vi "Jarvis main.vi"() -> ()   [LabVIEW 2017]
uses:
  SSL Referee Game Status.ctl
  Filters/Estimadores.ctl
  Control/SSL Data Control.ctl
  Control/SSL UDP Address.ctl
  Control/File Player.ctl
  Intel/Command Enum.ctl
  DrawTargets.ctl
  Util/Events/Events.ctl
  passTestStates.ctl
  SSL/SSL Field State.ctl
  SSL Detection Frame.ctl
  SSL Detection Robot.ctl
  <vilib>/Analysis/Matrix/Datatypes/RealMatrix.ctl
  SSL Detection Ball.ctl
  <extravilib>/ChannelInstances/Lossy Stream-a[.](u8)/Read With Abort.vi
  <extravilib>/ChannelInstances/Lossy Stream-t'SSL Referee Game Status.ctl'/Write With Abort.vi
  <extravilib>/ChannelInstances/Lossy Stream-c(a[.](c(c(dbl,dbl,dbl,dbl,dbl),c(dbl,dbl,dbl,dbl,dbl),c(dbl,dbl,dbl,dbl,dbl,u32),u32,u32)),t'Events.ctl')/Write With Abort.vi
  <extravilib>/ChannelInstances/Lossy Stream-c(t'AI Ball.ctl',a[.](c(c(dbl,dbl,dbl,dbl,dbl),c(dbl,dbl,dbl,dbl,dbl),c(dbl,dbl,dbl,dbl,dbl,u32),u32,u32)))/Write With Abort.vi
  <extravilib>/ChannelInstances/Lossy Stream-t'AI Input.ctl'/Read With Abort.vi
  <extravilib>/ChannelInstances/Lossy Stream-t'SSL Field State.ctl'/Write With Abort.vi
  <extravilib>/ChannelInstances/Lossy Stream-c(t'AI Ball.ctl',a[.](c(c(dbl,dbl,dbl,dbl,dbl),c(dbl,dbl,dbl,dbl,dbl),c(dbl,dbl,dbl,dbl,dbl,u32),u32,u32)))/Read With Abort.vi
  <extravilib>/ChannelInstances/Lossy Stream-c(a[.](c(c(dbl,dbl,dbl,dbl,dbl),c(dbl,dbl,dbl,dbl,dbl),c(dbl,dbl,dbl,dbl,dbl,u32),u32,u32)),t'Events.ctl')/Read With Abort.vi
  <extravilib>/ChannelInstances/Lossy Stream-a[.](i32)/Write With Abort.vi
  <extravilib>/ChannelInstances/Lossy Stream-t'SSL Referee Game Status.ctl'/Read With Abort.vi
  <extravilib>/ChannelInstances/Lossy Stream-t'SSL Field State.ctl'/Read With Abort.vi
  <extravilib>/ChannelInstances/Lossy Stream-t'AI Input.ctl'/Write With Abort.vi
  <extravilib>/ChannelInstances/Lossy Stream-a[.](u8)/EndpointRead.vi
  <extravilib>/ChannelInstances/Lossy Stream-t'SSL Referee Game Status.ctl'/Endpoint.vi
  <extravilib>/ChannelInstances/Lossy Stream-c(a[.](c(c(dbl,dbl,dbl,dbl,dbl),c(dbl,dbl,dbl,dbl,dbl),c(dbl,dbl,dbl,dbl,dbl,u32),u32,u32)),t'Events.ctl')/Endpoint.vi
  <extravilib>/ChannelInstances/Lossy Stream-c(t'AI Ball.ctl',a[.](c(c(dbl,dbl,dbl,dbl,dbl),c(dbl,dbl,dbl,dbl,dbl),c(dbl,dbl,dbl,dbl,dbl,u32),u32,u32)))/Endpoint.vi
  <extravilib>/ChannelInstances/Lossy Stream-t'AI Input.ctl'/EndpointRead.vi
  <extravilib>/ChannelInstances/Lossy Stream-t'SSL Field State.ctl'/Endpoint.vi
  <extravilib>/ChannelInstances/Lossy Stream-c(t'AI Ball.ctl',a[.](c(c(dbl,dbl,dbl,dbl,dbl),c(dbl,dbl,dbl,dbl,dbl),c(dbl,dbl,dbl,dbl,dbl,u32),u32,u32)))/EndpointRead.vi
  <extravilib>/ChannelInstances/Lossy Stream-c(a[.](c(c(dbl,dbl,dbl,dbl,dbl),c(dbl,dbl,dbl,dbl,dbl),c(dbl,dbl,dbl,dbl,dbl,u32),u32,u32)),t'Events.ctl')/EndpointRead.vi
  <extravilib>/ChannelInstances/Lossy Stream-a[.](i32)/Endpoint.vi
  <extravilib>/ChannelInstances/Lossy Stream-t'SSL Referee Game Status.ctl'/EndpointRead.vi
  <extravilib>/ChannelInstances/Lossy Stream-t'SSL Field State.ctl'/EndpointRead.vi
  <extravilib>/ChannelInstances/Lossy Stream-t'AI Input.ctl'/Endpoint.vi
  <extravilib>/ChannelInstances/Lossy Stream-t'AI Input.ctl'/Instantiate.vi
  <extravilib>/ChannelInstances/Lossy Stream-t'SSL Field State.ctl'/Instantiate.vi
  <extravilib>/ChannelInstances/Lossy Stream-t'AI Input.ctl'/)Channel.vi
  <resource>/ChannelSupport/_ChannelSupport/WaitIfNeeded.vi
  <extravilib>/ChannelInstances/Lossy Stream-c(t'AI Ball.ctl',a[.](c(c(dbl,dbl,dbl,dbl,dbl),c(dbl,dbl,dbl,dbl,dbl),c(dbl,dbl,dbl,dbl,dbl,u32),u32,u32)))/Instantiate.vi
  <extravilib>/ChannelInstances/Lossy Stream-c(a[.](c(c(dbl,dbl,dbl,dbl,dbl),c(dbl,dbl,dbl,dbl,dbl),c(dbl,dbl,dbl,dbl,dbl,u32),u32,u32)),t'Events.ctl')/Instantiate.vi
  <extravilib>/ChannelInstances/Lossy Stream-a[.](u8)/Instantiate.vi
  <extravilib>/ChannelInstances/Lossy Stream-a[.](u8)/)Channel.vi
  <extravilib>/ChannelInstances/Lossy Stream-c(t'AI Ball.ctl',a[.](c(c(dbl,dbl,dbl,dbl,dbl),c(dbl,dbl,dbl,dbl,dbl),c(dbl,dbl,dbl,dbl,dbl,u32),u32,u32)))/)Channel.vi
  <extravilib>/ChannelInstances/Lossy Stream-c(a[.](c(c(dbl,dbl,dbl,dbl,dbl),c(dbl,dbl,dbl,dbl,dbl),c(dbl,dbl,dbl,dbl,dbl,u32),u32,u32)),t'Events.ctl')/)Channel.vi
  <extravilib>/ChannelInstances/Lossy Stream-a[.](i32)/Instantiate.vi
  <extravilib>/ChannelInstances/Lossy Stream-t'SSL Referee Game Status.ctl'/Instantiate.vi
  <extravilib>/ChannelInstances/Lossy Stream-t'SSL Referee Game Status.ctl'/)Channel.vi
  SOS/passStateGlobalVariableResult.vi
  SOS/passTestAllResults.vi
  <extravilib>/ChannelInstances/Lossy Stream-a[.](i32)/)Channel.vi
  <extravilib>/ChannelInstances/Lossy Stream-t'SSL Field State.ctl'/)Channel.vi
  <extravilib>/ChannelInstances/Lossy Stream-t'SSL Referee Game Status.ctl'.lvlib
  <extravilib>/ChannelInstances/Lossy Stream-t'AI Input.ctl'.lvlib
  <extravilib>/ChannelInstances/Lossy Stream-t'SSL Field State.ctl'.lvlib
  <extravilib>/ChannelInstances/Lossy Stream-c(a[.](c(c(dbl,dbl,dbl,dbl,dbl),c(dbl,dbl,dbl,dbl,dbl),c(dbl,dbl,dbl,dbl,dbl,u32),u32,u32)),t'Events.ctl').lvlib
  <extravilib>/ChannelInstances/Lossy Stream-c(t'AI Ball.ctl',a[.](c(c(dbl,dbl,dbl,dbl,dbl),c(dbl,dbl,dbl,dbl,dbl),c(dbl,dbl,dbl,dbl,dbl,u32),u32,u32))).lvlib
  <extravilib>/ChannelInstances/Lossy Stream-a[.](i32).lvlib
  <extravilib>/ChannelInstances/Lossy Stream-a[.](u8).lvlib
  <vilib>/Analysis/Matrix/NI_Matrix.lvlib
panel:
  out "Comm FPS 5":dbl
  out "Comm FPS 4":dbl
  out "Comm FPS 3":dbl
  out "Comm FPS 2":dbl
  out "Events":T1={"Touch"=FALSE, "Ball out"=FALSE, "id touch"=0.0, "Ball out of \nVision"=FALSE, "Ball inside \nGoalie area"=FALSE, "Robot not responding"=FALSE, "Robots responding status"=[1.0, 1.0, 1.0, 1.0, 1.0, 1.0], "Enemy Ball \nPossession"=FALSE, "Pass State"=FALSE, "id end of pass"=0.0, "Kick"=FALSE, "Id ini Possession"=0.0, "Ball Possesion"=FALSE, "Id Possesion"=0.0}
  in  "Tab Control 2":T2(tab)
  out "2D Picture":picture
  out "Kick Error Histogram":cluster{dbl[], dbl[]}(graph)
  out "Goalie Error Histogram":cluster{dbl[], dbl[]}(graph)
  out "Heatmap by ID":picture
  in  "ID":i32
  in  "Enemy?":bool
  in  "Kalman Error\nID":i32
  out "Kalman Error Histogram":cluster{dbl[], dbl[]}(graph)
  out "Pass state":T3
  out "Ball out of the field":string
  out "Pass Intercepted":string
  out "Ball missed robot":string
  out "Need more force to pass":string
  out "Correct pass":string
  out "Too much force":string
  out "Number of goals":string
  in  "ID CSV Log":i32
  in  "Write?":bool
  in  "Erase file":bool
  in  "grid y":dbl=30.0 format="%#_13g"
  in  "grid x":dbl=45.0 format="%#_13g"
  in  "Draw Targets?":T4={"Attacker"=TRUE, "Striker"=TRUE, "Goalie"=TRUE, "Defender"=TRUE, "kick"=TRUE, "Est Ball"=TRUE, "Est Robot"=FALSE}
  in  "SSL Data":T5={"Modo"=TRUE, "SSL UDP RX"={"Port:"=10020, "Server IP:"="224.5.23.2", "Local IP:"="", "RX"=TRUE}, "RefBox UDP RX"={"Port:"=10003, "Server IP:"="224.5.23.1", "Local IP:"="", "RX"=TRUE}, "Reprodução de Arquivo"={"file path (use dialog)"=path "E:/Media/2016-07-01_cmdragons_immortals.log", "size (in bytes)"=0, "offset (in bytes)"=0, "Slide"=0.0, "Play"=FALSE, "Time Stamp"=timestamp(0 s since 1904-01-01), "Playing"=FALSE}, "SSL UDP SOS RX IA_State"={"Port:"=10025, "Server IP:"="224.5.23.2", "Local IP:"="", "RX"=TRUE}, "SSL UDP SOS RX  Enemy State"={"Port:"=10030, "Server IP:"="224.5.23.2", "Local IP:"="", "RX"=FALSE}} {"Reprodução de Arquivo"."Time Stamp" format="%<%.3X %x>T"; "Reprodução de Arquivo"."Slide" min=0 max=1 scale=0.0..1.0; "Reprodução de Arquivo"."offset (in bytes)" format="%.3p"; "Reprodução de Arquivo"."size (in bytes)" format="%.3p"}
  out "error out 3":errorcluster
  out "IA command":T8
  in  "ignora esquerda?":bool
  in  "ignora lado?":bool
  in  "Defense stretch":i32=300
  in  "Defense radius":i32=460
  in  "Estimador":T9=enum."Kalman"
  in  "Goalie":string(combo)="0"
  in  "Command":string(combo)="Auto"
  in  "Time":enum16{"Azul", "Amarelo"}(ring) caption="Enum"
  in  "Lado":enum16{"Esquerdo", "Direito"}(ring) caption="Enum"
  in  "Tab Control":enum32{"RX Info", "TX info", "AI Parameters"}(tab)
  out "Game Status":T10={"Stage"="Normal First Half Pre", "Command"="Stop", "Time Left"=0.0, "Yellow Team"="", "Blue Team"="", "Yellow Score"=0, "Blue Score"=0, "Yellow Red Cards"=0, "Blue Red Cards"=0, "Yellow Yellow Cards"=0, "Blue Yellow Cards"=0, "Yellow Timeouts Left"=0, "Blue Timeouts Left"=0, "Yellow Timeout Remaining"=0.0, "Blue Timeout Remaining"=0.0, "Yellow Goalie Id"=0, "Blue Goalie Id"=0, "Time"=timestamp(2082758400 s since 1904-01-01)} {"Time" format="%<%.3X %x>T"; "Blue Timeout Remaining" format="%<%M:%S>t"; "Yellow Timeout Remaining" format="%<%M:%S>t"; "Time Left" format="%<%M:%S>t"}
  in  "Jarvis to AI":bool=TRUE
  in  "Address:":string="127.0.0.1"
  in  "Port:":u16=10050
  out "Comm FPS":dbl
  # "UDP"
  # "LOG"
  # "Score"
  # "Red Cards"
  # "Yellow Cards"
  # "Timeouts Left"
  # "Timeout Remaining"
  # "Goalie ID"
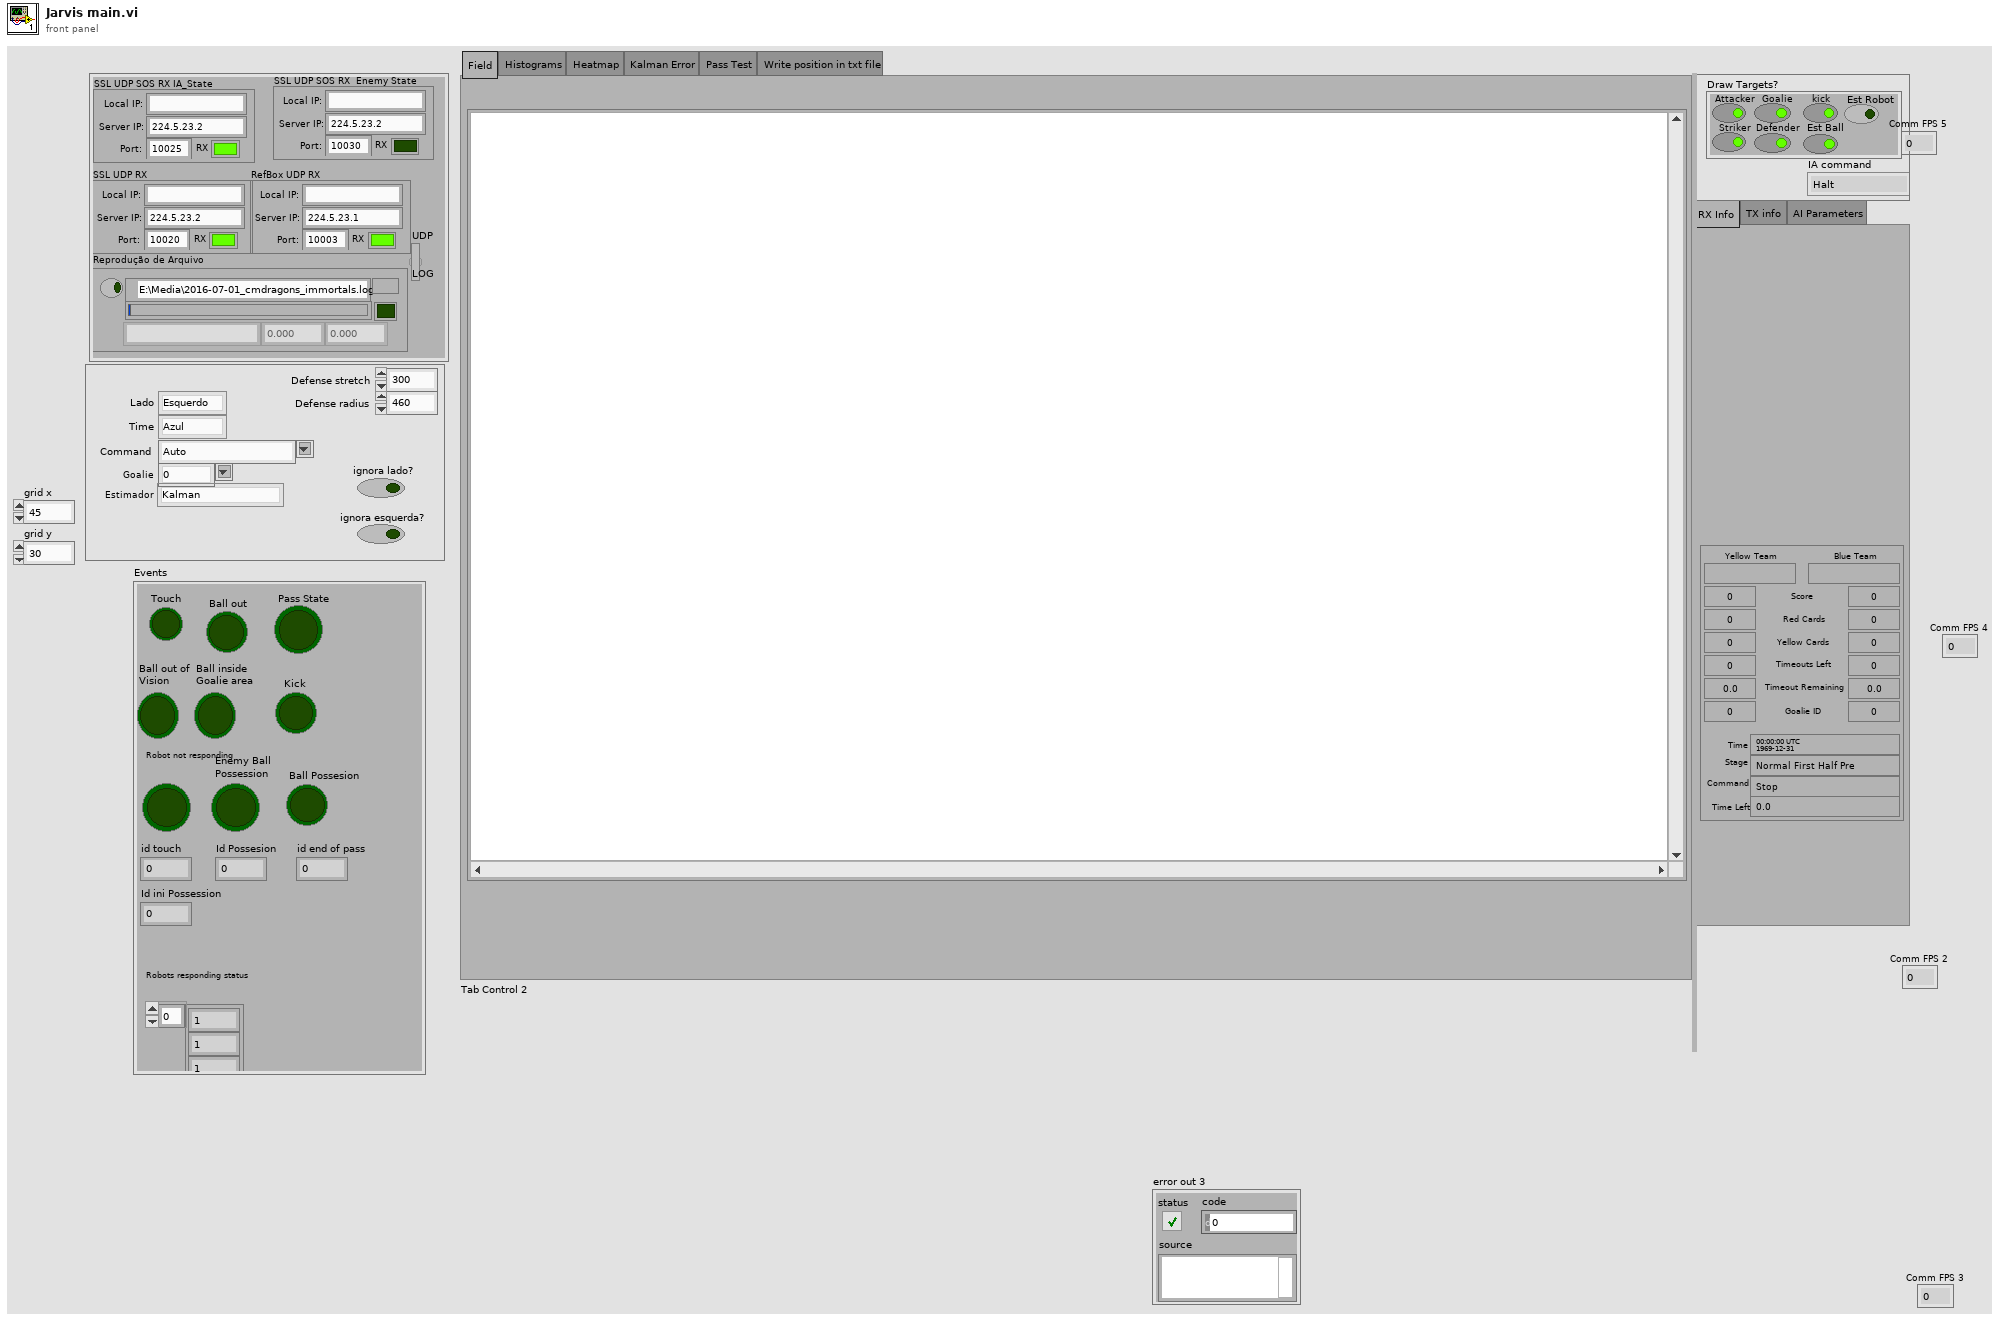
[diagram p1: front panel]
types:
  T1 = typedef "Events.ctl" = cluster{"Touch":bool, "Ball out":bool, "id touch":dbl, "Ball out of \nVision":bool, "Ball inside \nGoalie area":bool, "Robot not responding":bool, "Robots responding status":dbl[], "Enemy Ball \nPossession":bool, "Pass State":bool, "id end of pass":dbl, "Kick":bool, "Id ini Possession":dbl, "Ball Possesion":bool, "Id Possesion":dbl}
  T2 = enum32{"Field", "Histograms", "Heatmap", "Kalman Error", "Pass Test", "Write position in txt file"}
  T3 = typedef "passTestStates.ctl" = enum16{"Pass on the way", "Ball stops", "Pass intercepted", "Ball out of the field", "Ball missed robot", "Need more force to pass", "Too much force", "Correct pass", "Keep ball possesion", "Robot kicked the ball", "Waiting Kick", "Invalid: same robot", "Invalid: kicker ID 999", "Invalid: Receiver ID 999", "Invalid"}
  T4 = typedef "DrawTargets.ctl" = cluster{"Attacker":bool, "Striker":bool, "Goalie":bool, "Defender":bool, "kick":bool, "Est Ball":bool, "Est Robot":bool}
  T5 = typedef "SSL Data Control.ctl" = cluster{"Modo":bool, "SSL UDP RX":T6, "RefBox UDP RX":T6, "Reprodução de Arquivo":T7, "SSL UDP SOS RX IA_State":T6, "SSL UDP SOS RX  Enemy State":T6}
  T6 = typedef "SSL UDP Address.ctl" = cluster{"Port:":u16, "Server IP:":string, "Local IP:":string, "RX":bool}
  T7 = typedef "File Player.ctl" = cluster{"file path (use dialog)":path, "size (in bytes)":i64, "offset (in bytes)":i64, "Slide":sgl, "Play":bool, "Time Stamp":timestamp, "Playing":bool}
  T8 = typedef "Command Enum.ctl" = enum16{"Halt", "Stop", "Force Start", "PKA Normal Start", "Prepare Kickoff Ally", "PKE Normal Start", "Prepare Kickoff Enemy", "Prepare Penalty Ally", "PPA Normal Start", "Prepare Penalty Enemy", "PPE Normal Start", "Direct Free Enemy", "Direct Free Ally", "Indirect Free Enemy", "Indirect Free Ally", "Timeout Enemy", "Timeout Ally", "Goal Enemy", "Goal Ally", "Ball Placement Enemy", "Ball Placement Ally", "Normal Half Time", "Extra Time Break", "Extra Half Time", "None", "Post Game"}
  T9 = typedef "Estimadores.ctl" = enum16{"Nenhum", "Simples", "Kalman"}
  T10 = typedef "SSL Referee Game Status.ctl" = cluster{"Stage":string, "Command":string, "Time Left":dbl, "Yellow Team":string, "Blue Team":string, "Yellow Score":u32, "Blue Score":u32, "Yellow Red Cards":u32, "Blue Red Cards":u32, "Yellow Yellow Cards":u32, "Blue Yellow Cards":u32, "Yellow Timeouts Left":u32, "Blue Timeouts Left":u32, "Yellow Timeout Remaining":dbl, "Blue Timeout Remaining":dbl, "Yellow Goalie Id":u32, "Blue Goalie Id":u32, "Time":timestamp}
  T11 = typedef "Lossy Stream-a[.](u8).lvlib/)Channel.ctl" = refnum<queue>
  T12 = typedef "AI Ball.ctl" = cluster{"x":dbl, "y":dbl, "timestamp":timestamp, "Vel_x":dbl, "Vel_y":dbl, "Pos Bola Est":dbl[]}
  T13 = cluster{"Ball":T12, "Enemy_Robots":cluster{"Cinematics":cluster{"x":dbl, "y":dbl, "orientation":dbl, "est_vx":dbl, "est_vy":dbl}, "Destination":cluster{"dest_x":dbl, "dest_y":dbl, "dest_orientation":dbl, "dest_x_kick":dbl, "dest_y_kick":dbl}, "Commands":cluster{"v_tangent":dbl, "v_normal":dbl, "v_ang":dbl, "kick_x":dbl, "kick_z":dbl, "dribble":u32}, "id":u32, "function":u32}[]}
  T14 = typedef "Lossy Stream-c(t'AI Ball.ctl',a[.](c(c(dbl,dbl,dbl,dbl,dbl),c(dbl,dbl,dbl,dbl,dbl),c(dbl,dbl,dbl,dbl,dbl,u32),u32,u32))).lvlib/)Channel.ctl" = refnum<queue>
  T15 = typedef "SSL Field State.ctl" = cluster{"Detection Frame Out":T16, "Field Size Out":cluster{"line_width":u32, "field_length":u32, "field_width":u32, "boundary_width":u32, "referee_width":u32, "goal_width":u32, "goal_depth":u32, "goal_wall_width":u32, "center_circle_radius":u32, "defense_radius":u32, "defense_stretch":u32, "free_kick_from_defense_dist":u32, "penalty_spot_from_field_line_dist":u32, "penalty_line_from_spot_dist":u32}, "Received Time Stamp":timestamp}
  T16 = typedef "SSL Detection Frame.ctl" = cluster{"frame_number":u32, "t_capture":dbl, "t_sent":dbl, "camera_id":u32, "robots_yellow":T17[], "robots_blue":T17[], "balls":T19[], "Valid":bool, "Time Stamp":timestamp}
  T17 = typedef "SSL Detection Robot.ctl" = cluster{"x":sgl, "robot_id":u32, "confidence":sgl, "y":sgl, "orientation":sgl, "pixel_x":sgl, "pixel_y":sgl, "height":sgl, "Valid":bool, "Time Stamp":timestamp, "x_k|k":T18, "Pk|k":T18, "Previous Time Stamp":timestamp, "R":T18}
  T18 = typedef "NI_Matrix.lvlib/RealMatrix.ctl" = dbl[][]
  T19 = typedef "SSL Detection Ball.ctl" = cluster{"x":sgl, "area":u32, "confidence":sgl, "y":sgl, "z":sgl, "pixel_x":sgl, "pixel_y":sgl, "Valid":bool, "Time Stamp":timestamp, "x_k|k":T18, "Pk|k":T18, "Id":u32, "Previous Time Stamp":timestamp, "R":T18}
  T20 = cluster{"line_width":u32, "field_length":u32, "field_width":u32, "boundary_width":u32, "referee_width":u32, "goal_width":u32, "goal_depth":u32, "goal_wall_width":u32, "center_circle_radius":u32, "defense_radius":u32, "defense_stretch":u32, "free_kick_from_defense_dist":u32, "penalty_spot_from_field_line_dist":u32, "penalty_line_from_spot_dist":u32}
  T21 = typedef "Lossy Stream-t'SSL Field State.ctl'.lvlib/)Channel.ctl" = refnum<queue>
  T22 = cluster{"Our_Robots":cluster{"Cinematics":cluster{"x":dbl, "y":dbl, "orientation":dbl, "est_vx":dbl, "est_vy":dbl}, "Destination":cluster{"dest_x":dbl, "dest_y":dbl, "dest_orientation":dbl, "dest_x_kick":dbl, "dest_y_kick":dbl}, "Commands":cluster{"v_tangent":dbl, "v_normal":dbl, "v_ang":dbl, "kick_x":dbl, "kick_z":dbl, "dribble":u32}, "id":u32, "function":u32}[], "Events":T1}
  T23 = typedef "Lossy Stream-c(a[.](c(c(dbl,dbl,dbl,dbl,dbl),c(dbl,dbl,dbl,dbl,dbl),c(dbl,dbl,dbl,dbl,dbl,u32),u32,u32)),t'Events.ctl').lvlib/)Channel.ctl" = refnum<queue>
  T24 = typedef "SSL Referee.ctl" = cluster{"packet_\ntimestamp":u64, "stage":u64, "stage_time_left":i32, "command ":u64, "command_\ncounter ":u32, "command_\ntimestamp":u64, "yellow team info":T25, "blue team info":T25, "Point":cluster{"x":sgl, "y":sgl}}
  T25 = typedef "SSL Referee Team Info.ctl" = cluster{"name":string, "score":u32, "red_cards":u32, "yellow_cards_time":u32[], "yellow_cards":u32, "timeout":u32, "timeout_times":u32, "goalie":u32}
  T26 = typedef "Lossy Stream-t'SSL Referee Game Status.ctl'.lvlib/)Channel.ctl" = refnum<queue>
  T27 = typedef "AI Input.ctl" = cluster{"our_robots":T28[], "enemy_robots":T28[], "balls":T12[], "geometry":T31, "IA Judge":T32, "Received Timestamp":timestamp, "Events":T1}
  T28 = typedef "AI Robot.ctl" = cluster{"id":u32, "function":T29, "x":dbl, "y":dbl, "orientation":dbl, "v_tangent":dbl, "v_normal":dbl, "v_ang":dbl, "kick_x":dbl, "kick_z":dbl, "dribble":bool, "Timestamp":timestamp, "dest_x":dbl, "dest_y":dbl, "dest_orientation":dbl, "estimatives":cluster{"est_v_tangent":dbl, "est_v_normal":dbl, "est_vx":dbl, "est_vy":dbl, "Pos Robot Est":dbl[]}, "dest_x_kick":dbl, "dest_y_kick":dbl, "Gap Coord":dbl[], "States":T30}
  T29 = typedef "Functions Enum.ctl" = enum16{"Attacker", "Goalie", "Defender", "Striker", "Goto 0", "Dummy", "Kicker", "ZigZag"}
  T30 = typedef "AttackerStates.ctl" = enum16{"Pass", "GoToTangent", "BallGetting", "GoToKick", ""}
  T31 = typedef "Field Size.ctl" = cluster{"line_width":u32, "field_length":u32, "field_width":u32, "boundary_width":u32, "referee_width":u32, "goal_width":u32, "goal_depth":u32, "goal_wall_width":u32, "center_circle_radius":u32, "defense_radius":u32, "defense_stretch":u32, "free_kick_from_defense_dist":u32, "penalty_spot_from_field_line_dist":u32, "penalty_line_from_spot_dist":u32}
  T32 = typedef "AI Judge.ctl" = cluster{"stage":string, "command":string, "our_goalie_id":dbl, "enemy_goalie_id":dbl, "command enum":T8, "Time":enum16{"Azul", "Amarelo"}}
  T33 = typedef "Lossy Stream-a[.](i32).lvlib/)Channel.ctl" = refnum<queue>
  T34 = typedef "Lossy Stream-t'AI Input.ctl'.lvlib/)Channel.ctl" = refnum<queue>
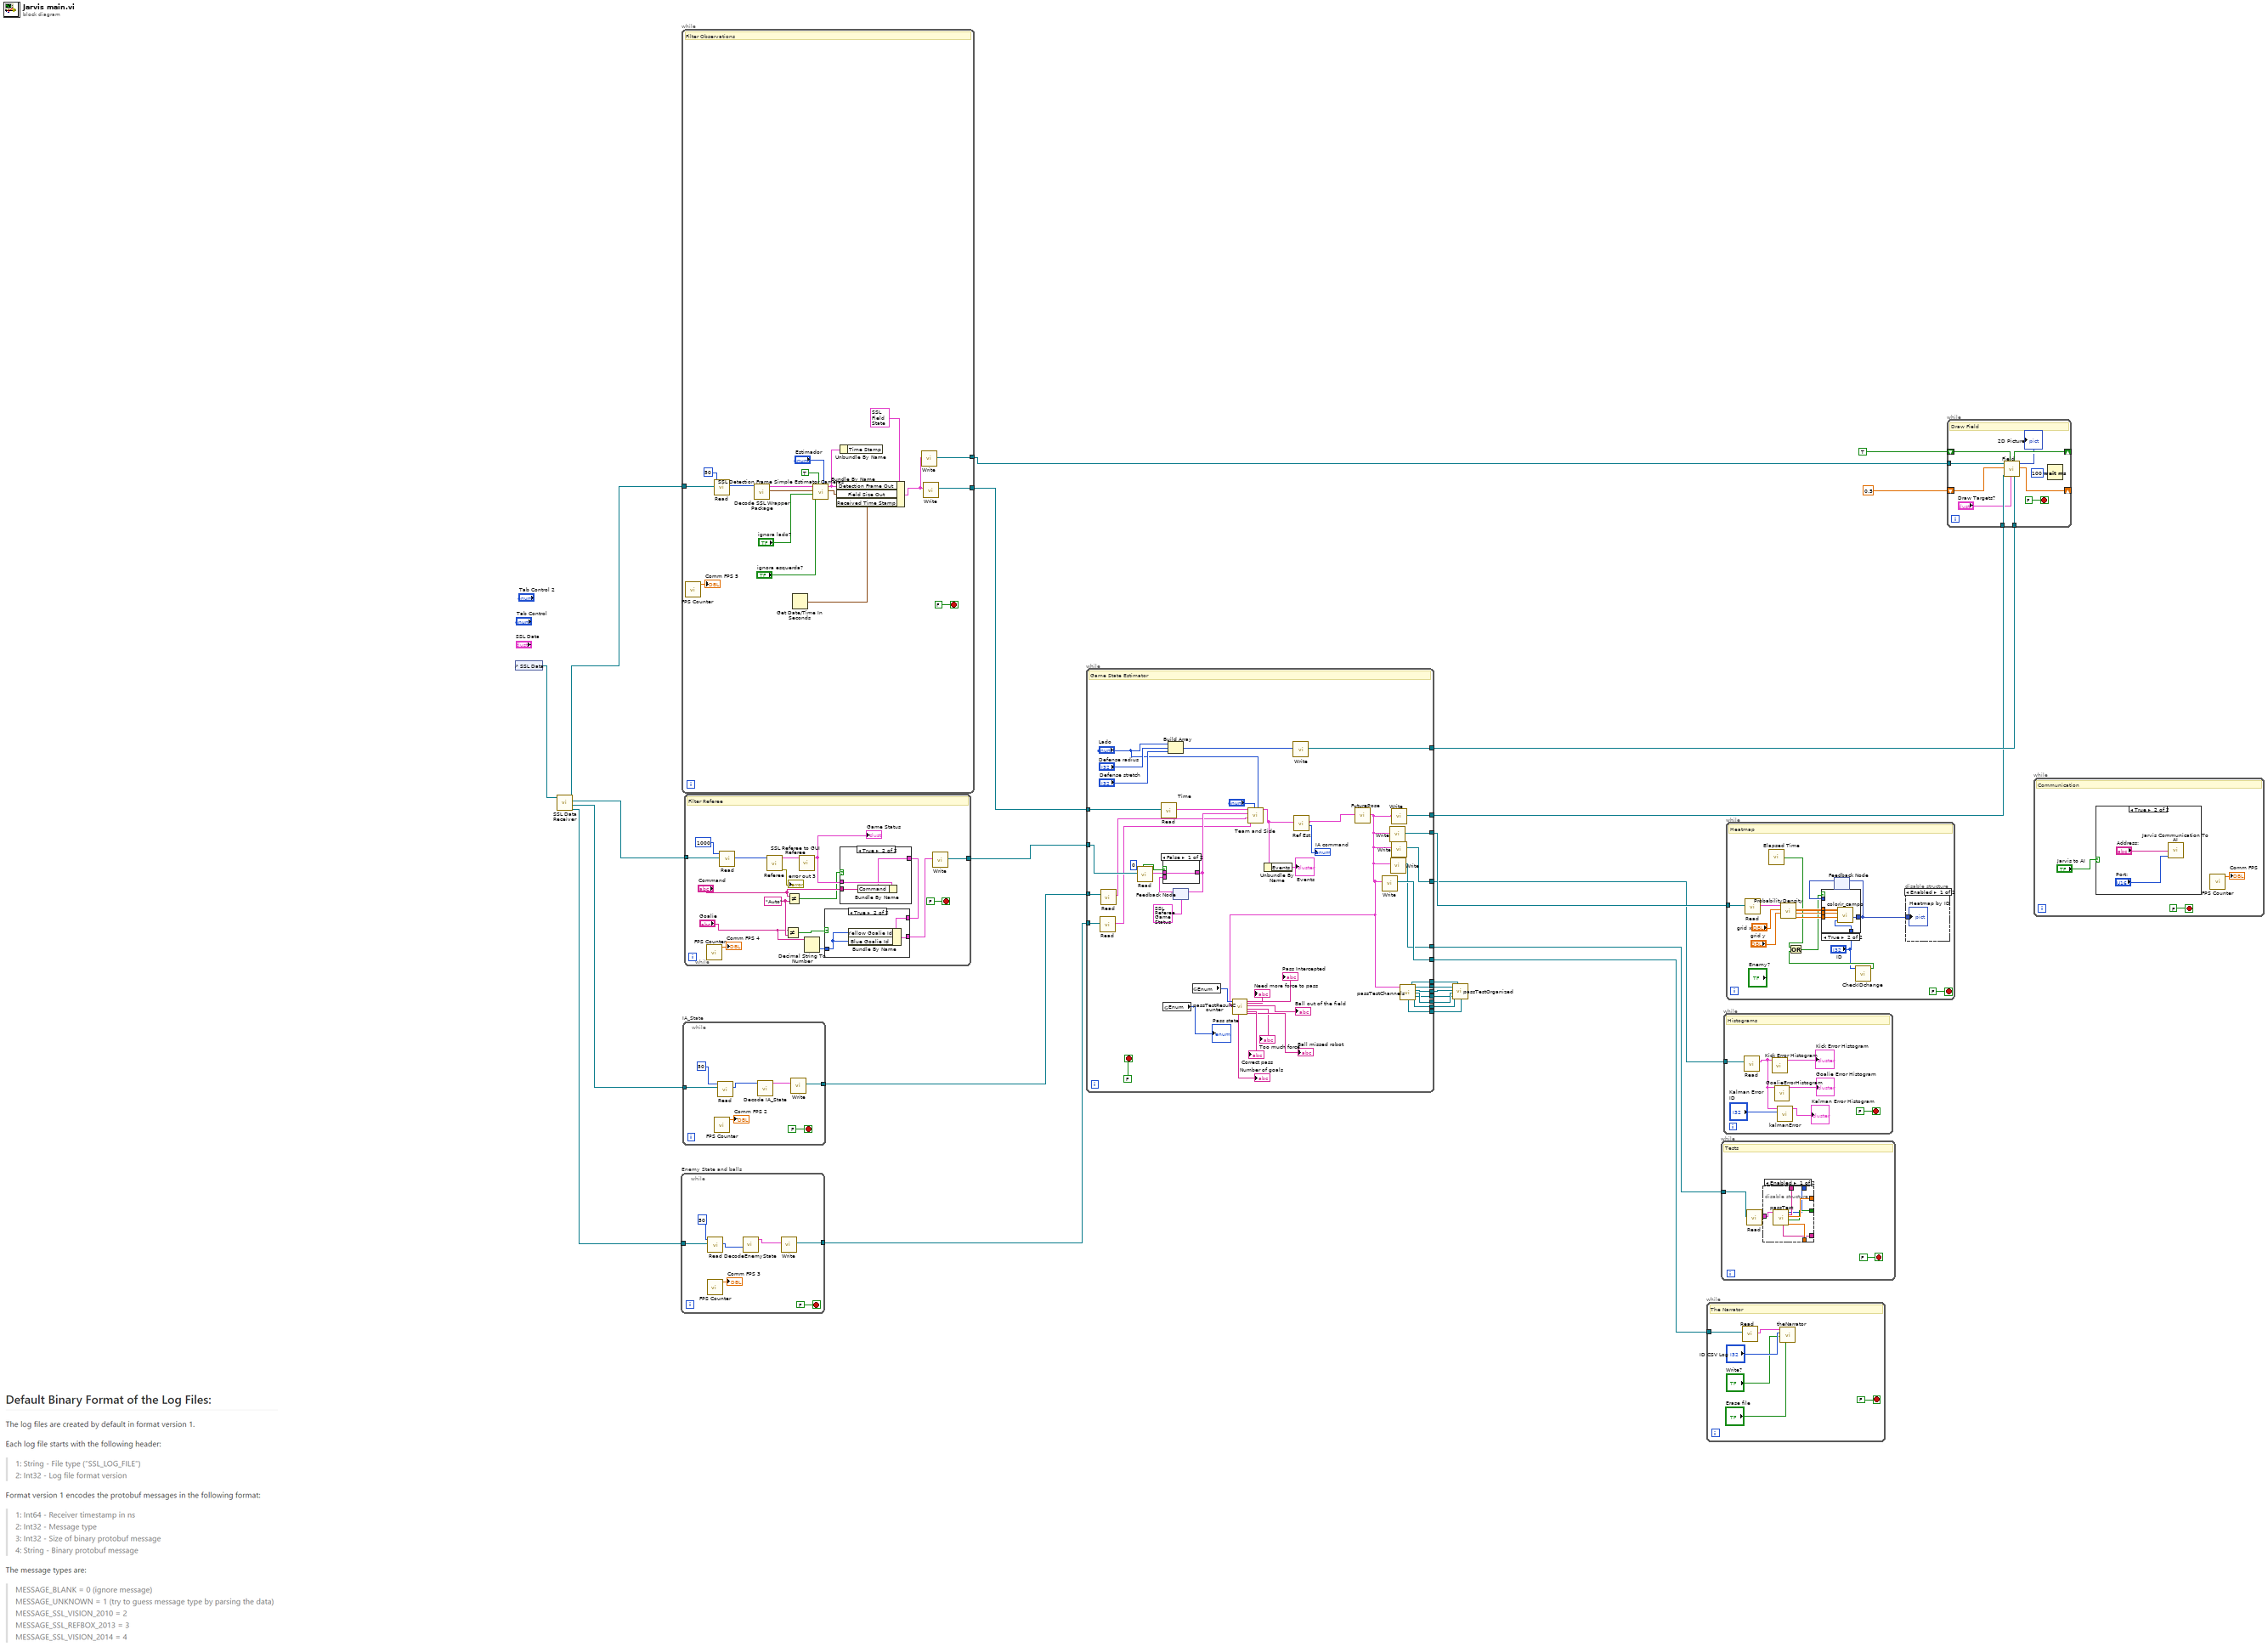
[diagram p0: block diagram]
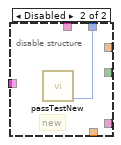
[diagram p6: hidden frame]
diagram:
  n1 = control-ref of="SSL Data"() -> (w16:refnum<vi>)
  n2 = call "SSL Data Receiver.vi"("SSL Data"=w16) -> ("Enemy_State"=w17:T11, "IA_State"=w18:T11, "SSL RefBox"=w20:T11, "SSL Vision"=w21:T11)  [unwired: 7 in]
  n3 = while "Enemy State and balls" {
    tunnel: w17 -> [w30]
    tunnel: [w27] -> w14
    stop <- FALSE stop-if-true
    n4 = call "FPS Counter.vi"() -> ("Numeric"=→"Comm FPS 3":dbl)  [unwired: 11 in]
    n5 = call <extravilib>:"Read.vi"("channel"=w30, "timeout in ms (-1)"=50) -> ("element"=w31:u8[])  [unwired: 4 in, 5 out]
    n6 = call "DecodeEnemyState.vi"("array"=w31) -> ("output cluster"=w28:T13)  [unwired: 8 in, 2 out]
    n7 = call <extravilib>:"Write.vi"("element"=w28) -> ("channel"=w27:T14)  [unwired: 8 in, 2 out]
  }
  n8 = while {
    tunnel: [w39] -> w2
    tunnel: [w44] -> w23
    tunnel: w21 -> [w36]
    stop <- FALSE stop-if-true
    # "Filter Observations"
    n9 = call "FPS Counter.vi"() -> ("Numeric"=→"Comm FPS 5":dbl)  [unwired: 11 in]
    n10 = call <extravilib>:"Read.vi"("channel"=w36, "timeout in ms (-1)"=50) -> ("element"=w35:u8[])  [unwired: 4 in, 5 out]
    n11 = call "Decode SSL Wrapper Package.vi"("unsigned byte array"=w35) -> ("Field Size"=w48:T20, "Detection Frame"=w49:T16)  [unwired: 7 in, 2 out]
    n12 = Get Date/Time In Seconds() -> (seconds since 1Jan1904=w46:timestamp)
    n13 = call "SSL Detection Frame Simple Estimator Cameras.vi"("Estimador"="Estimador", "Enable"=TRUE, "ignora esquerda?"="ignora esquerda?", "ignora lado?"="ignora lado?", "Field Size"=w48, "Detection Frame In"=w49) -> ("Field Size Out"=w45:T20, "Detection Frame Out"=w43:T16)  [unwired: 4 in]
    n14 = Bundle By Name(cluster=T15 {"Detection Frame Out"={"frame_number"=0, "t_capture"=0.0, "t_sent"=0.0, "camera_id"=0, "robots_yellow"=[], "robots_blue"=[], "balls"=[], "Valid"=FALSE, "Time Stamp"=timestamp(0 s since 1904-01-01)}, "Field Size Out"={"line_width"=0, "field_length"=0, "field_width"=0, "boundary_width"=0, "referee_width"=0, "goal_width"=0, "goal_depth"=0, "goal_wall_width"=0, "center_circle_radius"=0, "defense_radius"=0, "defense_stretch"=0, "free_kick_from_defense_dist"=0, "penalty_spot_from_field_line_dist"=0, "penalty_line_from_spot_dist"=0}, "Received Time Stamp"=timestamp(0 s since 1904-01-01)}, "Detection Frame Out"=w43, "Field Size Out"=w45, "Received Time Stamp"=w46) -> (w38:T15)
    n15 = Unbundle By Name(w43) -> ()  [unwired: 1 out]
    n16 = call <extravilib>:"Write.vi"("element"=w38) -> ("channel"=w39:T21)  [unwired: 8 in, 2 out]
    n17 = call <extravilib>:"Write.vi"("element"=w38) -> ("channel"=w44:T21)  [unwired: 8 in, 2 out]
  }
  n18 = while "IA_State" {
    tunnel: w18 -> [w56]
    tunnel: [w52] -> w15
    stop <- FALSE stop-if-true
    n19 = call "FPS Counter.vi"() -> ("Numeric"=→"Comm FPS 2":dbl)  [unwired: 11 in]
    n20 = call <extravilib>:"Read.vi"("channel"=w56, "timeout in ms (-1)"=50) -> ("element"=w54:u8[])  [unwired: 4 in, 5 out]
    n21 = call "Decode IA_State.vi"("array"=w54) -> ("output cluster"=w53:T22)  [unwired: 9 in, 1 out]
    n22 = call <extravilib>:"Write.vi"("element"=w53) -> ("channel"=w52:T23)  [unwired: 8 in, 2 out]
  }
  n23 = while {
    tunnel: w20 -> [w61]
    tunnel: [w71] -> w22
    stop <- FALSE stop-if-true
    w67 = "Auto" ("y")
    # "Filter Referee"
    n24 = call "FPS Counter.vi"() -> ("Numeric"=→"Comm FPS 4":dbl)  [unwired: 11 in]
    n25 = call <extravilib>:"Read.vi"("channel"=w61, "timeout in ms (-1)"=1000) -> ("element"=w60:u8[])  [unwired: 4 in, 5 out]
    n26 = call "Referee.vi"("element"=w60) -> ("output cluster"=w72:T24, "error out"=→"error out 3":errorcluster)  [unwired: 13 in]
    n27 = Not Equal?(x="Goalie", y=w67) -> (x != y?=w66:bool)
    n28 = Not Equal?(x="Command", y=w67) -> (x != y?=w68:bool)
    n29 = call "SSL Referee to GUI Referee.vi"("SSL Game Status"=w72) -> ("GUI Game Status"=w70:T10)  [unwired: 10 in]
    "Game Status" <- w70
    n30 = Decimal String To Number(string="Goalie") -> (number=w62:i32)  [unwired: 2 in, 1 out]
    n31 = case shown="True" w68 {
      tunnel: w70 -> [w79 w82]
      tunnel: [w79 w81] -> w65
      tunnel: "Command" -> [_ w80]
      frame False {
      }
      frame True {
        n32 = Bundle By Name(cluster=w82, "Command"=w80) -> (w81:T10)
      }
    }
    n33 = case shown="True" w66 {
      tunnel: w65 -> [w75 w78]
      tunnel: [w75 w77] -> w64
      tunnel: w62 -> [_ w76]
      frame False {
      }
      frame True {
        n34 = Bundle By Name(cluster=w78, "Yellow Goalie Id"=w76, "Blue Goalie Id"=w76) -> (w77:T10)
      }
    }
    n35 = call <extravilib>:"Write.vi"("element"=w64) -> ("channel"=w71:T26)  [unwired: 8 in, 2 out]
  }
  n36 = while {
    tunnel: w23 -> [w107]
    tunnel: w22 -> [w127]
    tunnel: [w109] -> w19
    tunnel: w15 -> [w115]
    tunnel: w14 -> [w114]
    tunnel: [w110] -> w13
    tunnel: [w105] -> w10
    tunnel: [w102] -> w11
    tunnel: [w101] -> w12
    tunnel: [w100] -> w9
    tunnel: [w99] -> w8
    tunnel: [w98] -> w7
    tunnel: [w97] -> w6
    tunnel: [w96] -> w5
    tunnel: [w95] -> w4
    tunnel: [w94] -> w3
    tunnel: [w84] -> w1
    stop <- FALSE stop-if-true
    # "Game State Estimator"
    n37 = call <extravilib>:"Read.vi"("channel"=w114) -> ("element"=w112:T13)  [unwired: 5 in, 5 out]
    n38 = call <extravilib>:"Read.vi"("channel"=w115) -> ("element"=w113:T22)  [unwired: 5 in, 5 out]
    n39 = call <extravilib>:"Read.vi"("channel"=w127, "timeout in ms (-1)"=0) -> ("element"=w124:T10, "timed out?"=w125:bool)  [unwired: 4 in, 4 out]
    n40 = call <extravilib>:"Read.vi"("channel"=w107) -> ("element"=w106:T15)  [unwired: 5 in, 5 out]
    n41 = global read "passStateGlobalVariableResult.vi" "Enum"() -> (→"Pass state":T3)
    n42 = Build Array("Lado", "Defense radius", "Defense stretch") -> (w108:i32[])
    n43 = feedback #1(T10 {"Stage"="First Half", "Command"="Stop", "Time Left"=0.0, "Yellow Team"="", "Blue Team"="", "Yellow Score"=0, "Blue Score"=0, "Yellow Red Cards"=0, "Blue Red Cards"=0, "Yellow Yellow Cards"=0, "Blue Yellow Cards"=0, "Yellow Timeouts Left"=0, "Blue Timeouts Left"=0, "Yellow Timeout Remaining"=0.0, "Blue Timeout Remaining"=0.0, "Yellow Goalie Id"=0, "Blue Goalie Id"=0, "Time"=timestamp(0 s since 1904-01-01)} ("element")) -> (w123:T10)
    n44 = case shown="False" w125 {
      tunnel: w124 -> [w129 _]
      tunnel: [w129 w130] -> w122
      tunnel: w123 -> [_ w130]
      frame False {
      }
      frame True {
      }
    }
    n45 = feedback-in #1(w122) -> ()
    n46 = global read "passTestAllResults.vi" "Enum"() -> (w86:T3)
    n47 = call "Team and Side.vi"("Lado"="Lado", "Time"="Time", "Enemy state and balls"=w112, "IA_State"=w113, "Game Status"=w122, "Field State Input"=w106) -> ("IA State"=w104:T27)  [unwired: 5 in]
    n48 = Unbundle By Name(w104) -> ("Events"=→"Events":T1)
    n49 = call <extravilib>:"Write.vi"("element"=w108) -> ("channel"=w109:T33)  [unwired: 8 in, 2 out]
    n50 = call "Ref Est.vi"("IA State Input"=w104) -> ("IA command"=→"IA command":T8, "IA State Output"=w111:T27)  [unwired: 9 in]
    n51 = call "FuturePose.vi"("IA State Input"=w111) -> ("output cluster"=w85:T27)  [unwired: 10 in]
    n52 = call "passTestResultCounter.vi"("IA State"=w85, "Pass state"=w86) -> ("Ball missed robot"=→"Ball missed robot":string, "Too much force"=→"Too much force":string, "Ball out of the field"=→"Ball out of the field":string, "Pass Intercepted"=→"Pass Intercepted":string, "Correct pass"=→"Correct pass":string, "Need more force to pass"=→"Need more force to pass":string, "Number of goals"=→"Number of goals":string)  [unwired: 3 in]
    n53 = call <extravilib>:"Write.vi"("element"=w85) -> ("channel"=w105:T34)  [unwired: 8 in, 2 out]
    n54 = call <extravilib>:"Write.vi"("element"=w85) -> ("channel"=w110:T34)  [unwired: 8 in, 2 out]
    n55 = call <extravilib>:"Write.vi"("element"=w85) -> ("channel"=w102:T34)  [unwired: 8 in, 2 out]
    n56 = call <extravilib>:"Write.vi"("element"=w85) -> ("channel"=w84:T34)  [unwired: 8 in, 2 out]
    n57 = call <extravilib>:"Write.vi"("element"=w85) -> ("channel"=w101:T34)  [unwired: 8 in, 2 out]
    n58 = call "passTestChannels.vi"("element"=w85) -> (3:"IA State"=w100:T34, 4:"IA State"=w99:T34, 6:"IA State"=w98:T34, 8:"IA State"=w97:T34, 10:"IA State"=w96:T34, 13:"IA State"=w94:T34, 15:"IA State"=w95:T34)  [unwired: 8 in]
  }
  n59 = call "passTestOrganized.vi"("IA State"=w8, 1:"IA state"=w9, 5:"IA state"=w7, 7:"IA state"=w6, 9:"IA state"=w5, 11:"IA state"=w4, 13:"IA state"=w3) -> ()  [unwired: 8 in, 1 out]
  n60 = while {
    tunnel: w10 -> [w135]
    stop <- FALSE stop-if-true
    # "The Narrator"
    n61 = call <extravilib>:"Read.vi"("channel"=w135) -> ("element"=w134:T27)  [unwired: 5 in, 5 out]
    n62 = call "theNarrator.vi"("Erase"="Erase file", "Write?"="Write?", "ID CSV Log"="ID CSV Log", "IA state"=w134) -> ()  [unwired: 8 in]
  }
  n63 = while {
    tunnel: w11 -> [w138]
    stop <- FALSE stop-if-true
    # "Tests"
    n64 = call <extravilib>:"Read.vi"("channel"=w138) -> ("element"=w137:T27)  [unwired: 5 in, 5 out]
    n65 = disable-structure shown="Enabled" {
      disable-tunnel: [w141 w147] -> _
      disable-tunnel: [w146 _] -> _
      disable-tunnel: [w145 _] -> _
      disable-tunnel: [w144 _] -> _
      disable-tunnel: [w143 _] -> _
      disable-tunnel: [w142 _] -> _
      disable-tunnel: w137 -> [w140 _]
      frame Enabled {
        n66 = call "passTest.vi"("IA state"=w140) -> ("ID Kicker Robot"=w144:dbl, "Pass finished"=w145:bool, "ID Receiving Robot"=w146:dbl, "Pass state"=w141:T3, "Last pass"=w143:string, "Last lines"=w142:string[])  [unwired: 5 in]
      }
      frame Disabled {
        # "new"
        n67 = call "passTestNew.vi"() -> ("Enum 2"=w147:T3, "Initial channel"=w148:T34)  [unwired: 10 in]
      }
    }
  }
  n68 = while {
    tunnel: w12 -> [w154]
    stop <- FALSE stop-if-true
    # "Histograms"
    n69 = call <extravilib>:"Read.vi"("channel"=w154) -> ("element"=w151:T27)  [unwired: 5 in, 5 out]
    n70 = call "Kick Error Histogram.vi"("IA state"=w151) -> ("Kick Error Histogram"=→"Kick Error Histogram":cluster{dbl[], dbl[]})  [unwired: 10 in]
    n71 = call "GoalieErrorHistogram.vi"("IA state"=w151) -> ("Goalie Error Histogram"=→"Goalie Error Histogram":cluster{dbl[], dbl[]})  [unwired: 10 in]
    n72 = call "kalmanError.vi"("Kalman Error ID"="Kalman Error\nID", "IA state"=w151) -> ("Kalman Error Histogram"=→"Kalman Error Histogram":cluster{dbl[], dbl[]})  [unwired: 9 in]
  }
  n73 = while {
    tunnel: w13 -> [w162]
    stop <- FALSE stop-if-true
    # "Heatmap"
    n74 = call <extravilib>:"Read.vi"("channel"=w162) -> ("element"=w163:T27)  [unwired: 5 in, 5 out]
    n75 = call "Elapsed Time"() -> ("Time has Elapsed"=w158:bool)  [unwired: 12 in, 7 out]
    n76 = call "ProbabilityDensity.vi"("grid y"="grid y", "grid x"="grid x", "IA state"=w163) -> ("grid y out"=w164:dbl, "grid x out"=w165:dbl, "3D Probability Matrix"=w166:dbl[][][])  [unwired: 6 in]
    n77 = feedback #2() -> (w160:picture)  [unwired: 1 in]
    n78 = call "CheckIDchange.vi"("ID"="ID") -> ("ID change"=w159:bool)  [unwired: 10 in]
    n79 = Or(x=w158, y=w159) -> (x .or. y?=w157:bool)
    n80 = case shown="True" w157 {
      tunnel: w166 -> [_ w175]
      tunnel: w165 -> [_ w174]
      tunnel: w164 -> [_ w173]
      tunnel: [w170 w172] -> w161
      tunnel: "ID" -> [_ w171]
      tunnel: w160 -> [w170 _]
      frame False {
      }
      frame True {
        n81 = call "colorir_campo.vi"("ID"=w171, "grid y"=w173, "grid x"=w174, "3D Probability Matrix"=w175) -> ("campo colorido"=w172:picture)  [unwired: 7 in]
      }
    }
    n82 = feedback-in #2(w161) -> ()
    n83 = disable-structure shown="Enabled" {
      disable-tunnel: w161 -> [w176 _]
      frame Enabled {
        "Heatmap by ID" <- w176
      }
      frame Disabled {
      }
    }
  }
  n84 = while {
    shift-right: [w186] -> _
    shift-left: 0.5 ("New Scale") -> [w181]
    shift-right: [w185] -> _
    shift-left: TRUE ("AutoScale Out") -> [w184]
    tunnel: w1 -> [w182]
    tunnel: w19 -> [w180]
    tunnel: w2 -> [w177]
    stop <- FALSE stop-if-true
    # "Draw Field"
    n85 = call "Field.vi"("channel 2"=w180, "Draw Targets?"="Draw Targets?", "AutoScale"=w184, "channel for IA State"=w182, "Scale mm/pixel"=w181, "channel"=w177) -> ("Scale Out"=w186:dbl, "2D Picture"=→"2D Picture":picture, "AutoScale Out"=w185:bool)  [unwired: 3 in]
    n86 = Wait (ms)(milliseconds to wait=u32 100) -> ()  [unwired: 1 out]
  }
  n87 = while {
    stop <- FALSE stop-if-true
    # "Communication"
    n88 = case shown="True" "Jarvis to AI" {
      frame False {
      }
      frame True {
        n89 = call "Jarvis Communication To AI.vi"("Port:"="Port:", "SSL Vision Address:"="Address:") -> ()  [unwired: 10 in]
      }
    }
    n90 = call "FPS Counter.vi"() -> ("Numeric"=→"Comm FPS":dbl)  [unwired: 11 in]
  }
